vi "Main_04b.vi"() -> ()   [LabVIEW 2020]
uses:
  3a1e2d73-e658-461c-8538-171ed0141bef.vi
panel:
  out "sum 2":i16
  in  "Puzzle":string="31-31,32-40\n26-92,13-91\n9-90,29-91\n72-72,25-73\n28-79,79-79\n52-77,53-53\n17-54,17-54\n11-47,4-10\n1-96,1-97\n38-99,39-63\n19-54,18-53\n1-73,1-73\n17-34,18-34\n93-93,25-94\n96-98,7-95\n58-97,73-98\n7-64,8-64\n87-91,67-90\n42-78,77-85\n24-96,24-97\n71-78,72-97\n5-28,27-29\n19-86,86-90\n19-85,20-20\n64-65,1-64\n28-78,27-81\n79-91,80-95\n32-89,32-82\n3-96,2-4\n70-83,15-70\n5-90,8-91\n16-60,16-61\n38-97,39-90\n25-56,6-55\n12-14,13-13\n11-95,11-96\n13-16,12-22\n15-29,14-72\n68-88,67-69\n23-95,94-97\n63-77,62-64\n19-69,20-85\n23-63,61-62\n7-47,6-47\n39-86,39-86\n98-99,4-98\n4-6,5-88\n41-89,88-89\n14-95,96-98\n6-62,3-62\n1-68,6-68\n25-90,40-90\n11-81,10-12\n2-91,1-91\n35-62,27-61\n14-28,14-28\n13-78,14-79\n51-52,46-52\n6-77,77-78\n98-99,50-98\n7-23,24-85\n38-56,38-62\n96-99,1-97\n32-32,31-31\n5-89,4-6\n22-84,21-85\n14-40,39-89\n40-91,40-91\n3-6,4-60\n48-59,60-60\n2-92,2-92\n34-35,7-34\n32-64,33-64\n36-56,36-55\n95-96,44-96\n91-99,37-92\n10-98,11-96\n24-68,69-94\n98-99,37-98\n99-99,6-87\n11-90,11-12\n76-87,36-77\n19-97,10-99\n47-77,78-93\n96-96,21-96\n50-97,99-99\n3-50,2-81\n18-69,19-69\n17-92,16-16\n18-72,19-72\n1-76,5-77\n14-97,98-99\n28-90,19-89\n19-47,47-48\n10-97,9-97\n11-96,11-85\n20-22,20-97\n1-94,1-95\n49-52,48-53\n3-3,3-34\n12-97,85-96\n49-84,48-84\n3-89,89-90\n68-96,41-96\n69-80,2-65\n16-81,16-81\n1-96,95-99\n49-99,49-94\n28-92,91-95\n2-95,1-99\n12-30,8-31\n21-68,26-69\n6-31,2-31\n49-66,49-65\n55-67,55-68\n21-50,20-44\n14-42,15-43\n70-89,70-89\n3-99,1-3\n7-86,6-37\n58-71,68-71\n55-83,55-82\n61-99,11-99\n83-83,3-84\n25-82,25-81\n14-48,15-54\n97-98,13-96\n25-63,63-63\n4-81,37-82\n12-98,98-98\n31-34,33-56\n3-83,1-82\n33-99,99-99\n96-99,39-97\n82-84,43-77\n95-99,1-96\n83-84,6-83\n58-60,58-58\n51-92,92-93\n93-93,33-93\n1-93,92-97\n16-16,16-31\n10-55,54-55\n56-64,63-70\n18-88,10-19\n55-95,5-95\n62-77,48-61\n3-65,56-65\n54-55,55-56\n22-70,23-70\n18-91,18-18\n91-98,2-99\n9-56,8-56\n84-92,17-83\n98-98,25-99\n22-63,66-84\n4-50,2-5\n12-13,12-49\n30-85,31-79\n57-83,57-87\n13-79,13-79\n30-38,17-87\n64-65,5-64\n99-99,29-99\n28-75,7-27\n3-79,3-67\n10-90,24-89\n10-53,83-91\n39-74,35-39\n52-78,53-78\n2-87,3-95\n58-68,57-68\n6-32,31-51\n18-36,18-35\n3-99,3-99\n8-81,7-80\n50-53,51-52\n91-92,84-92\n19-91,5-18\n40-68,68-69\n30-90,52-91\n20-27,19-26\n98-99,99-99\n27-58,28-58\n61-61,45-62\n67-75,60-77\n69-70,68-72\n1-96,4-93\n2-95,38-96\n56-57,11-56\n54-84,6-53\n65-85,5-66\n22-84,21-84\n50-64,51-53\n7-75,74-81\n34-69,34-70\n35-35,6-35\n8-96,69-96\n13-98,13-97\n80-80,55-81\n16-62,6-98\n2-87,63-87\n84-91,7-92\n3-3,4-98\n3-80,52-80\n80-94,11-79\n2-95,1-71\n31-96,95-95\n9-65,64-65\n61-69,60-97\n2-99,2-98\n18-73,19-21\n80-80,80-82\n47-70,47-71\n13-30,23-30\n16-41,17-41\n3-13,12-79\n72-75,73-87\n13-13,13-81\n29-74,30-73\n24-43,7-42\n1-93,92-93\n4-47,4-93\n8-10,9-96\n2-87,5-88\n51-61,50-64\n60-64,60-63\n26-66,27-73\n13-85,14-86\n42-43,42-92\n45-72,44-44\n83-83,84-99\n3-5,6-97\n10-92,10-10\n43-69,44-69\n49-50,15-50\n4-91,4-91\n51-52,20-51\n7-84,1-96\n6-76,5-76\n15-19,14-14\n57-68,46-69\n80-80,3-81\n4-93,7-92\n37-40,38-41\n8-49,16-49\n6-86,86-87\n71-85,71-85\n35-68,69-96\n57-96,2-56\n13-33,5-32\n14-97,14-97\n83-98,60-99\n4-24,10-25\n1-84,2-84\n75-86,70-74\n22-79,1-78\n94-94,10-93\n6-70,7-70\n25-56,16-20\n2-87,1-88\n50-52,51-92\n2-68,3-42\n3-93,92-92\n8-97,96-96\n90-93,77-94\n61-98,6-99\n30-47,16-47\n27-92,26-26\n18-32,19-32\n23-76,19-21\n8-43,23-44\n9-93,10-93\n64-85,84-86\n2-88,88-89\n51-77,32-78\n53-83,25-52\n74-97,74-99\n99-99,7-98\n3-96,3-96\n67-67,68-69\n3-96,2-99\n18-95,17-19\n41-43,42-59\n3-5,5-5\n4-98,3-98\n41-69,70-88\n21-90,20-89\n76-78,77-81\n12-47,46-46\n33-85,34-84\n12-14,13-91\n46-59,45-59\n73-79,72-94\n7-18,6-8\n35-94,94-95\n15-18,15-18\n22-94,23-68\n15-16,15-81\n71-71,39-72\n61-61,11-62\n38-69,84-98\n76-80,76-79\n8-71,71-72\n27-94,28-71\n5-34,5-69\n48-62,35-61\n30-30,31-95\n45-96,95-99\n27-86,28-87\n72-72,44-72\n3-90,2-96\n31-98,30-71\n77-77,8-78\n19-99,18-20\n96-96,88-97\n10-30,7-8\n46-94,46-94\n9-34,33-96\n34-79,7-78\n31-77,32-76\n25-50,26-49\n37-70,36-38\n31-58,32-58\n12-97,12-98\n85-91,7-86\n57-77,4-78\n18-64,64-64\n73-74,72-74\n1-42,1-2\n30-99,37-98\n35-97,31-97\n17-57,57-58\n65-86,19-85\n27-95,50-97\n16-75,3-74\n44-87,86-94\n4-52,3-8\n31-96,95-95\n13-39,1-40\n29-95,71-95\n8-93,6-6\n1-97,2-98\n2-9,10-90\n22-24,19-23\n12-95,31-87\n1-77,7-78\n10-83,3-9\n60-88,60-87\n46-76,41-75\n21-57,20-57\n70-86,70-99\n46-56,55-72\n4-80,14-20\n14-55,13-71\n4-21,3-22\n2-91,2-92\n10-54,9-55\n1-3,2-98\n2-94,1-97\n3-89,3-4\n3-91,10-90\n11-13,10-68\n70-79,69-71\n42-77,42-77\n16-97,1-97\n18-82,82-86\n8-51,8-60\n21-70,20-70\n4-93,5-92\n46-46,6-45\n9-88,8-88\n26-92,15-91\n16-17,16-66\n58-65,7-65\n19-21,20-54\n48-93,48-93\n42-86,43-85\n28-44,28-44\n13-13,14-97\n10-72,73-73\n94-94,15-95\n44-67,26-66\n16-97,15-94\n74-74,9-75\n8-43,1-51\n33-58,34-57\n25-29,54-79\n21-77,29-76\n30-31,30-93\n88-96,42-87\n11-92,10-93\n25-72,2-73\n1-99,4-99\n33-56,33-80\n16-93,15-94\n36-39,34-38\n31-68,31-31\n20-89,88-90\n87-87,43-87\n12-14,11-14\n5-27,5-28\n28-70,71-71\n16-98,25-97\n13-89,12-12\n27-33,10-34\n97-99,54-95\n12-84,85-89\n39-58,40-57\n43-44,43-54\n92-94,93-95\n47-48,47-87\n10-31,9-30\n5-96,4-97\n67-70,67-71\n20-52,53-72\n44-65,38-66\n34-55,34-94\n1-98,6-89\n4-83,57-82\n94-95,4-93\n57-58,17-58\n8-38,5-9\n5-88,87-87\n17-76,75-77\n5-9,5-10\n31-36,28-31\n50-50,44-51\n19-89,19-89\n34-54,35-96\n54-60,32-64\n56-78,56-77\n39-39,39-39\n21-22,20-21\n52-76,51-53\n62-89,63-71\n40-85,40-70\n5-15,16-90\n42-83,41-46\n40-98,4-98\n29-94,28-54\n62-92,91-98\n8-94,9-93\n83-88,51-88\n4-60,7-60\n41-72,41-49\n31-57,51-56\n49-99,49-94\n79-79,10-80\n21-86,57-87\n42-44,23-43\n7-94,8-94\n24-32,24-33\n32-51,39-52\n12-28,27-82\n50-63,50-97\n58-64,64-64\n72-72,73-77\n51-65,51-51\n41-98,42-98\n97-98,1-97\n5-76,5-75\n83-93,42-92\n87-87,2-88\n26-41,26-27\n68-71,67-70\n61-62,36-62\n6-66,1-31\n57-73,15-72\n11-97,96-97\n4-99,4-98\n22-54,22-54\n18-43,43-43\n2-39,3-7\n24-91,99-99\n98-98,48-97\n3-70,3-71\n71-85,81-84\n93-98,2-92\n79-86,9-80\n30-61,60-83\n31-37,23-36\n25-95,26-95\n43-56,42-69\n18-28,5-27\n11-87,12-86\n58-99,59-97\n3-3,3-70\n31-41,17-30\n14-27,14-15\n2-70,3-94\n2-93,1-93\n38-90,39-79\n57-99,1-79\n70-95,70-78\n24-89,23-88\n4-84,19-83\n46-70,5-47\n10-70,71-73\n13-95,14-95\n48-52,49-52\n20-22,21-21\n88-88,1-88\n39-84,45-83\n28-75,28-75\n17-17,17-95\n3-98,97-97\n9-21,9-97\n28-37,27-34\n32-47,32-46\n13-28,27-72\n43-65,5-43\n22-48,47-48\n8-90,91-95\n51-53,10-52\n34-65,30-65\n1-98,1-2\n65-79,13-79\n74-74,13-75\n31-33,32-99\n4-95,38-94\n10-90,90-91\n62-62,4-61\n14-24,24-46\n4-85,10-84\n15-83,14-83\n1-85,3-86\n12-12,13-13\n15-89,14-90\n72-94,23-73\n11-69,8-68\n20-90,16-17\n5-95,32-96\n49-71,49-91\n22-89,22-89\n4-43,5-5\n51-98,15-97\n85-85,28-85\n18-61,18-81\n88-89,56-88\n71-79,72-79\n3-84,19-85\n18-18,19-85\n15-15,4-15\n46-71,44-71\n56-88,7-89\n37-50,36-51\n84-84,55-83\n14-27,15-26\n74-76,22-75\n77-99,77-95\n13-44,20-45\n6-95,12-96\n11-41,10-12\n10-76,17-77\n8-84,9-85\n14-64,13-15\n5-82,3-3\n43-53,42-44\n14-74,2-75\n12-97,12-98\n59-93,93-94\n17-81,15-82\n87-91,24-92\n8-84,9-84\n20-94,93-99\n46-97,97-98\n87-97,52-97\n2-90,3-91\n36-74,38-73\n55-59,55-55\n49-69,48-59\n54-62,54-96\n49-74,10-48\n27-78,26-26\n31-31,29-30\n2-76,1-90\n10-98,7-97\n14-15,14-93\n24-95,95-98\n13-23,22-23\n6-66,5-5\n85-86,66-86\n3-97,96-99\n1-93,1-90\n27-77,27-28\n51-64,51-51\n13-83,6-83\n40-54,53-54\n3-94,1-4\n15-29,15-28\n6-83,84-95\n62-62,8-63\n12-76,13-76\n3-7,5-7\n10-93,11-98\n28-28,28-63\n11-34,10-98\n6-8,7-49\n8-22,6-34\n29-47,29-49\n97-97,53-80\n20-99,21-75\n3-56,7-57\n43-63,43-64\n3-99,2-99\n24-99,24-25\n40-41,40-59\n60-63,60-60\n13-87,3-14\n70-88,25-88\n39-96,96-97\n11-53,12-52\n35-48,48-49\n11-53,9-25\n65-75,74-91\n74-80,80-80\n10-12,12-13\n46-73,74-84\n4-80,81-99\n4-84,83-91\n6-86,40-79\n46-82,22-81\n15-40,16-39\n5-86,45-93\n4-31,3-5\n40-84,31-83\n6-88,5-88\n8-79,12-80\n10-94,9-95\n81-81,23-81\n9-28,1-9\n47-99,46-83\n24-41,24-85\n10-67,9-35\n28-61,16-61\n6-6,7-71\n42-87,10-99\n97-97,2-97\n38-43,37-44\n15-86,15-87\n3-93,3-4\n85-86,84-87\n3-94,1-3\n32-47,47-47\n47-47,28-48\n4-97,4-98\n11-18,37-61\n31-38,30-38\n1-37,3-37\n23-60,61-99\n93-98,37-94\n8-97,9-97\n59-95,59-59\n81-87,13-80\n6-97,4-16\n15-27,27-73\n12-95,4-96\n54-96,22-55\n72-76,71-81\n5-94,6-92\n24-78,25-78\n55-64,52-63\n51-65,59-64\n32-87,32-58\n7-58,34-58\n29-83,29-82\n3-94,3-95\n84-84,71-85\n4-98,3-5\n17-36,18-37\n38-49,37-50\n14-61,94-99\n61-82,96-96\n25-98,98-99\n63-78,64-64\n43-49,42-50\n43-47,43-47\n14-62,23-63\n7-97,9-64\n49-82,49-90\n2-59,2-60\n53-85,53-86\n1-99,56-99\n26-92,26-60\n70-83,2-52\n54-55,54-85\n37-71,70-77\n87-91,15-92\n11-61,12-61\n9-9,7-10\n22-53,20-54\n88-89,1-88\n9-80,79-91\n43-85,43-59\n34-88,35-87\n9-98,24-97\n80-85,7-79\n9-38,38-39\n56-56,56-67\n79-90,79-89\n29-61,60-61\n1-95,1-96\n60-66,60-66\n41-75,74-74\n18-55,54-77\n4-98,3-97\n5-14,2-13\n9-51,9-55\n26-62,35-63\n85-97,84-96\n2-99,98-98\n67-94,67-94\n10-18,17-96\n12-99,13-13\n8-99,10-99\n20-28,21-27\n77-87,58-78\n38-51,38-59\n19-90,19-59\n24-98,37-74\n49-88,28-89\n18-85,84-85\n36-48,37-48\n70-92,91-93\n45-50,45-91\n82-93,44-50\n1-97,97-99\n45-58,44-59\n4-21,20-78\n56-83,57-57\n92-92,25-92\n33-36,35-35\n17-86,22-74\n12-86,86-87\n36-41,2-40\n34-34,35-35\n12-95,94-98\n88-89,32-99\n13-90,12-31\n3-90,1-1\n9-96,9-99\n8-60,13-61\n91-96,97-97\n19-58,18-20\n4-4,4-76\n2-57,2-75\n97-99,18-93\n15-37,38-86\n55-94,54-87\n15-35,16-94\n15-57,59-97\n14-90,14-91\n25-53,54-54\n87-97,86-97\n8-13,48-75\n5-80,3-3\n65-79,65-78\n1-73,72-73\n67-69,46-67\n50-67,49-67\n23-59,22-59\n2-27,1-96\n14-33,1-32\n30-82,16-30\n8-18,14-19\n30-30,27-30\n99-99,11-56\n25-26,25-38\n61-66,65-65\n44-77,93-97\n36-36,37-93\n11-45,10-10\n32-57,31-56\n98-99,41-96\n98-99,11-99\n6-8,7-79\n18-87,45-87\n22-84,22-92\n3-91,9-81\n5-78,6-78\n1-83,82-95\n54-61,54-61\n67-86,66-94\n17-85,17-86\n41-41,41-66\n57-68,14-67\n6-7,7-96\n10-96,72-98\n21-73,20-74\n35-98,9-97\n98-98,12-99\n6-48,5-96\n18-96,97-98\n19-21,20-52\n10-71,1-72\n2-35,2-2\n13-85,85-86\n29-81,81-82\n5-77,78-96\n40-41,28-41\n2-92,1-91\n7-81,28-82\n38-72,37-39\n58-85,25-85\n3-43,2-4\n30-58,31-79\n73-76,22-74\n43-73,44-74\n47-83,46-82\n64-92,63-69\n49-90,90-90\n11-98,11-97\n45-83,44-64\n18-65,38-65\n7-97,6-98\n9-67,11-77\n10-99,9-98\n11-41,10-58\n91-91,20-44\n2-99,2-98\n69-77,70-81\n45-73,46-55\n16-17,16-17\n13-76,75-81\n9-38,9-18\n42-64,3-41\n2-8,7-54\n53-58,28-59\n86-87,2-86\n93-93,13-94\n99-99,17-98\n55-63,60-60\n9-54,8-54\n89-95,94-95\n30-87,86-86\n14-16,15-96\n9-90,8-8\n41-95,40-94\n75-91,88-91\n9-13,8-10\n5-93,93-93\n19-41,19-41\n58-65,57-59\n56-99,55-70\n76-76,3-68\n98-98,46-92\n73-89,74-76\n78-93,26-78\n26-26,27-77\n57-76,75-75\n64-82,64-98\n64-91,21-80\n30-65,64-64\n43-43,43-87\n29-93,28-92\n94-95,13-95\n23-95,22-86\n18-85,84-84\n23-34,22-99\n82-84,77-84\n11-30,11-31\n6-34,33-34\n19-59,19-60\n4-66,65-72\n57-75,24-58\n26-55,34-54\n23-62,17-61\n1-89,3-92\n20-38,20-37\n10-98,10-11\n5-93,58-87\n89-90,62-90\n69-70,38-69\n36-63,62-63\n38-49,39-92\n86-87,22-87\n99-99,52-78\n16-99,16-92\n62-64,63-64\n87-88,69-87\n55-78,69-78\n5-15,15-72\n52-60,16-61\n4-97,1-96\n2-85,19-85\n5-10,1-22\n37-81,31-82\n21-91,12-90\n70-71,37-70\n64-64,65-92\n40-93,94-98\n38-84,83-85\n44-97,44-98\n31-31,10-31\n28-96,27-27\n32-79,35-78\n72-93,8-88\n7-77,7-58\n8-93,2-8\n5-91,28-90\n2-96,1-96\n52-56,51-54\n8-85,6-85\n4-84,6-49\n9-98,2-8\n61-97,46-60\n95-96,66-94\n98-98,86-99\n27-28,27-97\n54-85,55-86\n91-91,35-90\n4-89,10-88\n6-97,5-80\n34-57,35-37\n6-98,6-98\n12-67,31-68\n35-93,34-36\n11-60,39-61\n66-81,40-96\n57-57,8-56\n15-79,10-80\n78-79,27-79\n45-62,46-63\n14-35,35-71\n12-49,11-13\n51-67,67-67\n67-68,54-68\n55-93,13-41\n22-91,21-23\n92-95,88-96\n82-94,82-94\n99-99,2-97\n6-46,6-46\n39-75,1-40\n8-54,54-55\n78-93,77-93\n67-95,95-95\n2-4,3-98\n17-95,94-94\n36-51,42-50\n1-95,1-94\n67-96,67-95\n7-78,3-77\n18-48,17-47\n76-96,5-95\n45-45,21-46\n48-76,47-76\n36-38,33-38\n17-33,13-70\n78-93,78-78\n3-50,2-50\n8-8,8-84\n33-97,33-96\n51-53,52-87\n21-42,22-42\n98-99,2-98\n8-99,8-97\n41-51,41-51\n20-75,68-74\n2-98,98-99\n46-95,68-88\n16-69,68-97\n41-96,95-97\n1-98,1-98\n35-93,35-97\n54-66,1-97\n29-98,29-97\n44-44,44-67\n7-69,69-69\n3-74,73-73\n8-78,9-75\n43-51,51-52\n13-49,48-48\n42-76,3-76\n16-50,9-55\n62-71,62-71\n79-98,7-66\n43-58,58-58\n25-30,25-54\n2-17,16-27\n88-99,15-87\n33-94,94-94\n9-11,10-43\n38-97,39-95\n17-58,18-57\n25-97,17-62\n9-19,10-26\n87-88,86-87\n23-58,22-59\n49-96,49-49\n64-81,31-70\n3-85,2-86\n10-10,9-28\n9-51,5-9\n49-57,48-57\n1-65,3-66\n54-70,70-71\n2-61,1-60\n90-98,57-91"
  in  "Example":string="2-4,6-8\n2-3,4-5\n5-7,7-9\n2-8,3-7\n6-6,4-6\n2-6,4-8"
  # "--- Part Two ---\nIt seems like there is still quite a bit of duplicate work planned. Instead, the Elves would like to know the number of pairs that overlap at all.\n\nIn the above example, the first two pairs (2-4,6-8 and 2-3,4-5) don't overlap, while the remaining four pairs (5-7,7-9, 2-8,3-7, 6-6,4-6, and 2-6,4-8) do overlap:\n\n5-7,7-9 overlaps in a single section, 7.\n2-8,3-7 overlaps all of the sections 3 through 7.\n6-6,4-6 overlaps in a single section, 6.\n2-6,4-8 overlaps in sections 4, 5, and 6.\nSo, in this example, the number of overlapping assignment pairs is 4.\n\nIn how many assignment pairs do the ranges overlap?"
  # "876"
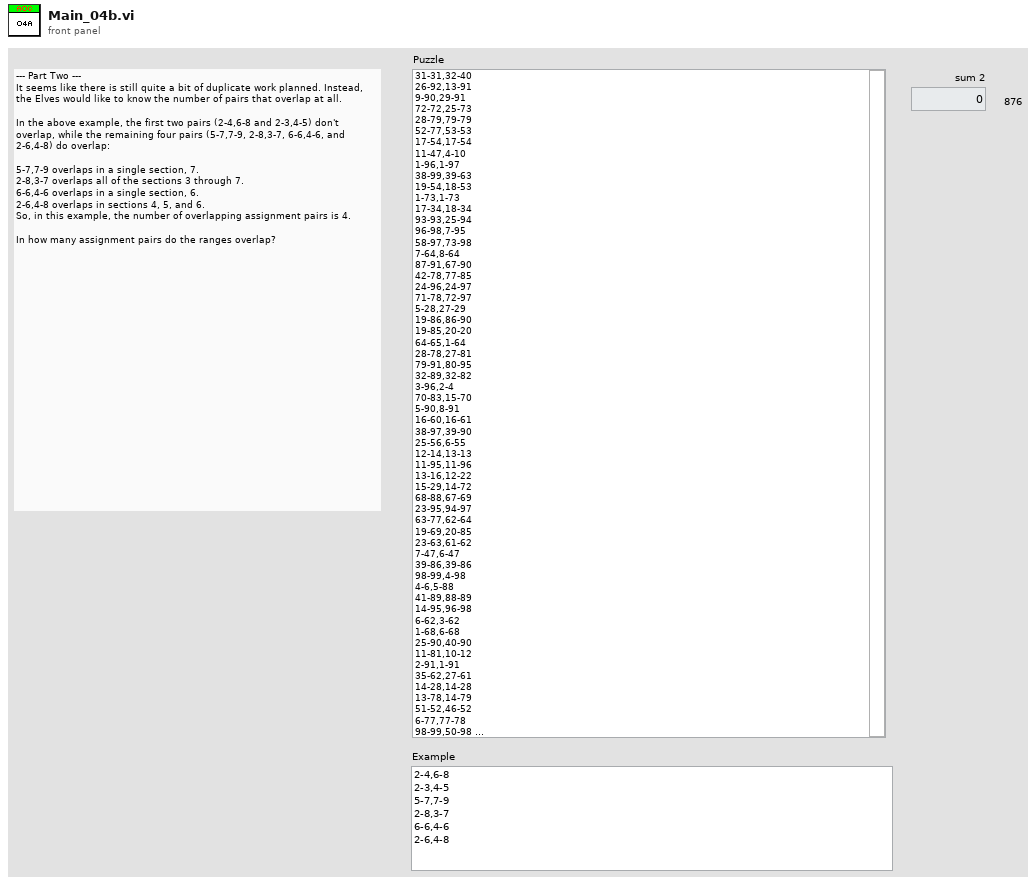
[diagram p1: front panel]
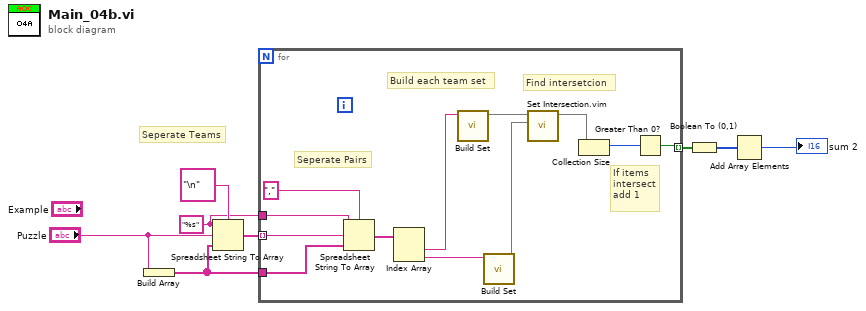
[diagram p0: block diagram]
diagram:
  w5 = "%s" ("format string")
  # "Seperate Teams"
  n1 = Build Array("Puzzle") -> (w7:string[])
  n2 = Spreadsheet String To Array(delimiter (Tab)="\n", format string=w5, spreadsheet string="Puzzle", array type (2D Dbl)=w7) -> (array=w4:string[])
  n3 = for {
    tunnel: w7 -> [w16]
    tunnel: w5 -> [w18]
    tunnel: w4 -> [w17] mode=indexing
    tunnel: [w9] -> w3 mode=indexing
    # "If items\nintersect\nadd 1"
    # "Find intersetcion"
    # "Build each team set"
    # "Seperate Pairs"
    n4 = Spreadsheet String To Array(delimiter (Tab)=",", format string=w18, spreadsheet string=w17, array type (2D Dbl)=w16) -> (array=w15:string[])
    n5 = Index Array(array=w15) -> (element #1=w13:string, element #2=w12:string)  [unwired: 2 in]
    n6 = call "Build Set.vi"("Example"=w13) -> ("Set"=w14:set{i32})  [unwired: 10 in]
    n7 = call "Build Set.vi"("Example"=w12) -> ("Set"=w20:set{i32})  [unwired: 10 in]
    n8 = call "Set Intersection.vim"("set 2"=w20, "set 1"=w14) -> ("intersection"=w11:set{i32})  [unwired: 9 in]
    n9 = Collection Size(1:w11) -> (0:w10:i32)
    n10 = Greater Than 0?(x=w10) -> (x > 0?=w9:bool)
  }
  n11 = Boolean To (0,1)(Boolean=w3) -> (0, 1=w2:i16[])
  n12 = Add Array Elements(numeric array=w2) -> (sum=→"sum 2":i16)
